vi "makeFrame.vi"(8 "error in (no error)":errorcluster, 9 "Data":u8[](array[numeric]) format="%.0x", 11 "RTU in":refnum<class "RTU.lvclass">) -> (0 "error out":errorcluster, 2 "Frame":string, 3 "RTU out":refnum<class "RTU.lvclass">)   [LabVIEW 2015, in "ModBUS.lvlib" / "RTU.lvclass"]
uses:
  RTU.lvclass
panel:
  # "11 03 006B 0003"
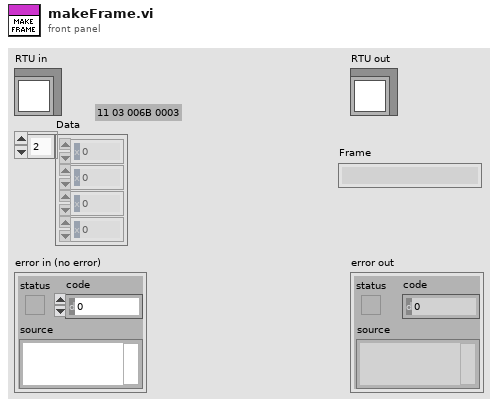
[diagram p1: front panel]
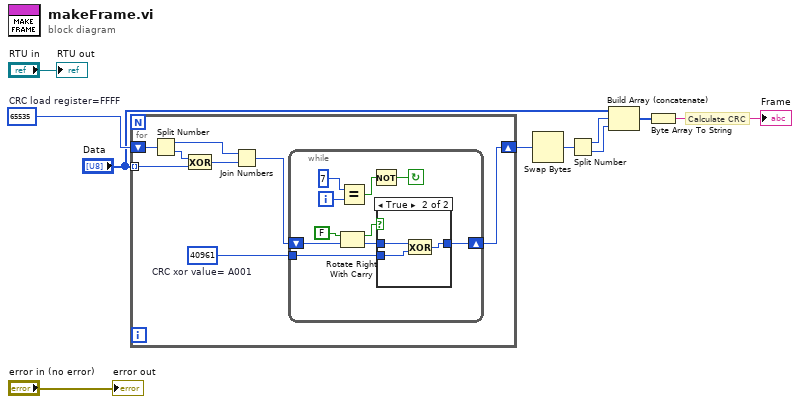
[diagram p0: block diagram]
diagram:
  w9 = u16 65535  # CRC load register=FFFF
  # "Calculate CRC"
  n1 = for {
    tunnel: "Data" -> [w17] mode=indexing
    shift-right: [w16] -> w8
    shift-left: w9 -> [w18]
    w11 = u16 40961  # CRC xor value= A001
    n2 = Split Number(x=w18) -> (hi(x)=w12:u8, lo(x)=w14:u8)
    n3 = Exclusive Or(1:w17, 2:w14) -> (0:w13:u8)
    n4 = Join Numbers(hi=w12, lo=w13) -> ((hi.lo)=w15:u16)
    n5 = while {
      shift-left: w15 -> [w24]
      shift-right: [w25] -> w16
      tunnel: w11 -> [w27]
      i -> [w22]
      stop <- w26 continue-if-true
      n6 = Rotate Right With Carry(2:w24, 3:FALSE) -> (0:w19:u16, 1:w21:bool)
      n7 = Equal?(x=7, y=w22) -> (x = y?=w20:bool)
      n8 = Not(x=w20) -> (.not. x?=w26:bool)
      n9 = case shown="True" w21 {
        tunnel: w19 -> [w29 w32]
        tunnel: w27 -> [_ w31]
        tunnel: [w29 w30] -> w25
        frame False {
        }
        frame True {
          n10 = Exclusive Or(1:w31, 2:w32) -> (0:w30:u16)
        }
      }
    }
  }
  n11 = Swap Bytes(anything=w8) -> (byte swapped=w7:u16)
  n12 = Split Number(x=w7) -> (hi(x)=w6:u8, lo(x)=w5:u8)
  n13 = Build Array (concatenate)("Data", w6, w5) -> (w4:u8[])
  n14 = Byte Array To String(unsigned byte array=w4) -> (string=→"Frame":string)
  "error out" <- "error in (no error)"
  "RTU out" <- "RTU in"
